vi "sidereal_time.vi"(0 "TimeStamp [UT]":timestamp format="%<%H:%M:%S%6u\n%Y/%m/%d>T", 1 "ee":dbl) -> (2 "gst":dbl[unit])   [LabVIEW 2009]
uses:
  lib/novas-dll.dll
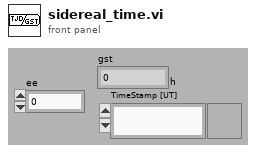
[diagram p1: front panel]
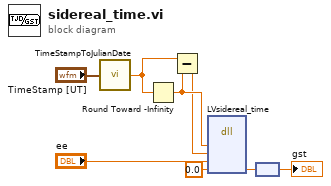
[diagram p0: block diagram]
diagram:
  n1 = call "TimeStampToJulianDate.vi"("TimeStamp [UT]"="TimeStamp [UT]") -> ("JulianDay"=w3:ext)
  n2 = Round Toward -Infinity(1:w3) -> (0:w2:ext)
  n3 = Subtract(x=w3, y=w2) -> (x-y=w1:ext)
  n4 = dll-call lib="C:/Ohana/LV2009/OhanaOS-LV81/Instruments/Novas/lib/novas-dll.dll" fn="LVsidereal_time"("jd_high"=w2, "jd_low"=w1, "ee"="ee", "gst"=0.0) -> ("gst"=w7:dbl)  [unwired: 4 in, 5 out]
  n5 = node(w7) -> (→"gst":dbl[unit])
